vi "Registration with Fourier Mellin Transform.vi"() -> ()   [LabVIEW 2023]
uses:
  <vilib>/vision/NI_Vision_Development_Module.lvlib
panel:
  out "max value (\"Similarity)":sgl
  in  "Images":u16(ring) items=["Shift1-1_Shift1-2", "Shift2-1_Shift2-2"]
  out "DIFF Image":T1(plugin-control)
  out "Inv FFT":T1(plugin-control)
  out "Image 2":T1(plugin-control)
  out "Image 1":T1(plugin-control)
  out "Y Shift":i32
  out "X Shift":i32
  # "Images Registration using Fourier-Mellin Transform"
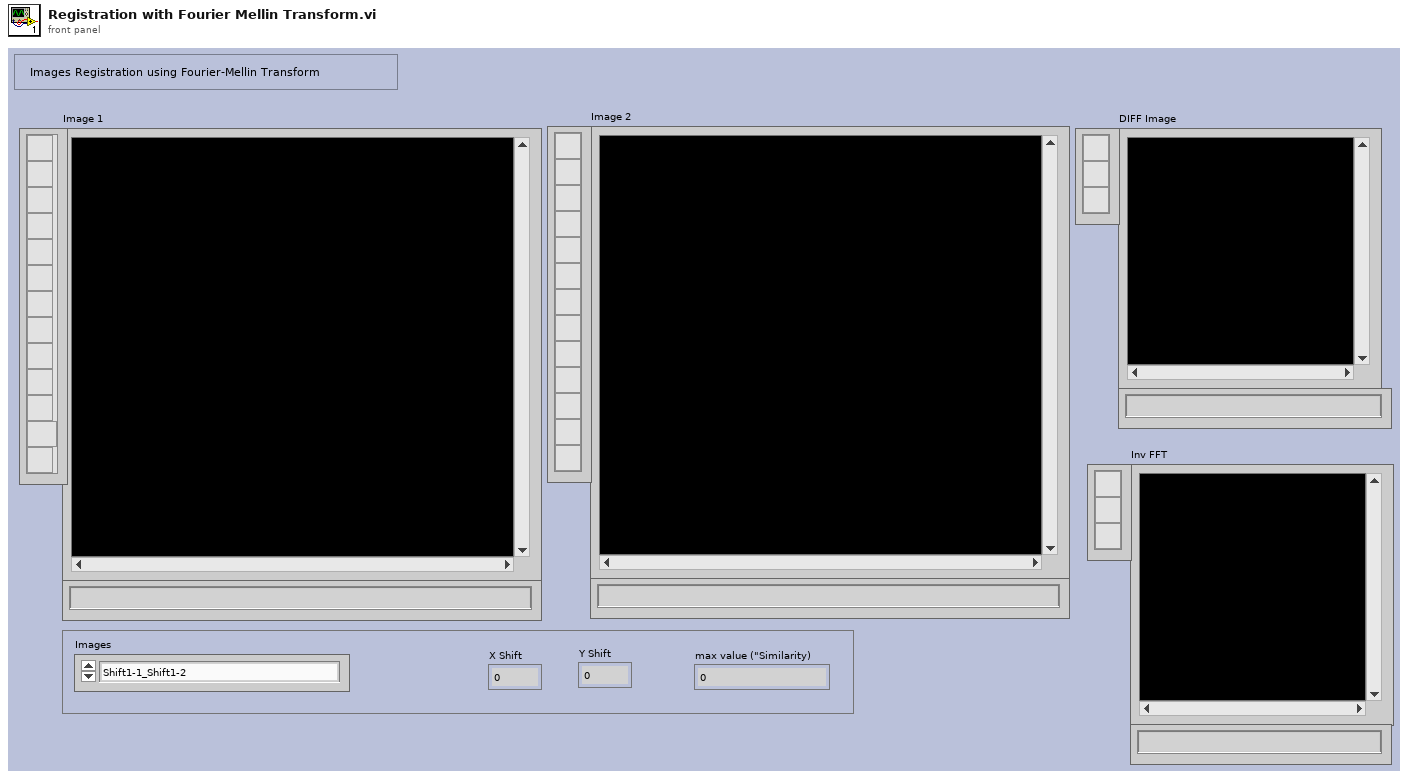
[diagram p1: front panel]
types:
  T1 = typedef "IMAQ Image.ctl" = refnum<image>
  T2 = cluster{"Global Rectangle":i32[], "Contours":cluster{"Contour Type":u32, "ROI Type":u32, "Points":i32[]}[]}
  T3 = typedef "Image Type" = u32
  T4 = typedef "ROI Descriptor" = cluster{"Global Rectangle":i32[], "Contours":cluster{"ID":enum32{"External", "Internal"}, "Type":u32, "Coordinates":i32[]}[]}
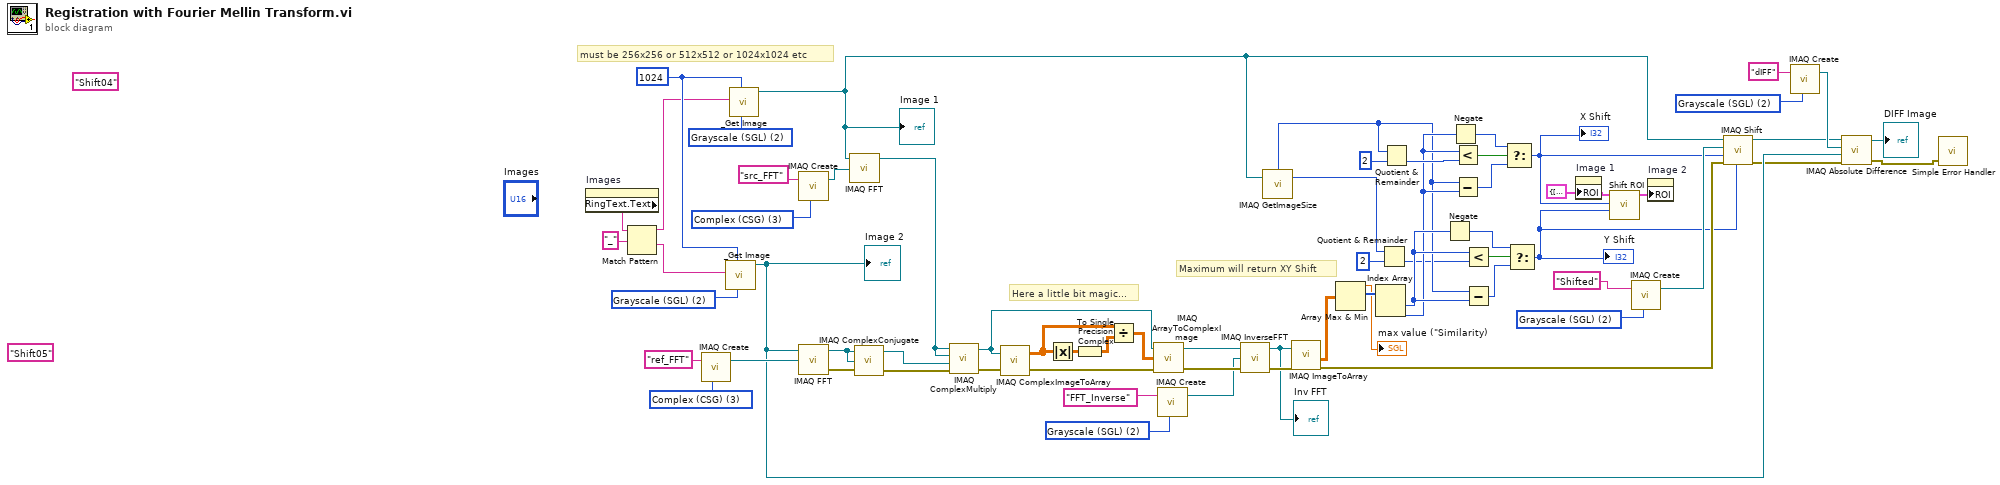
[diagram p0: block diagram]
diagram:
  w5 = T2 {"Global Rectangle"=[344, 290, 717, 642], "Contours"=[{"Contour Type"=0, "ROI Type"=4, "Points"=[404, 335, 668, 593]}, {"Contour Type"=0, "ROI Type"=2, "Points"=[536, 290, 536, 641]}, {"Contour Type"=0, "ROI Type"=2, "Points"=[344, 464, 716, 464]}]} ("ROI")
  w16 = T3 3 items=["Grayscale (U8)", "Grayscale (I16)", "Grayscale (SGL)", "Complex (CSG)", "RGB (U32)", "HSL (U32)", "RGB (U64)", "Grayscale (U16)"] ("Image Type")
  w31 = T3 2 items=["Grayscale (U8)", "Grayscale (I16)", "Grayscale (SGL)", "Complex (CSG)", "RGB (U32)", "HSL (U32)", "RGB (U64)", "Grayscale (U16)"] ("Image Type")
  w32 = T3 3 items=["Grayscale (U8)", "Grayscale (I16)", "Grayscale (SGL)", "Complex (CSG)", "RGB (U32)", "HSL (U32)", "RGB (U64)", "Grayscale (U16)"] ("Image Type")
  w33 = T3 2 items=["Grayscale (U8)", "Grayscale (I16)", "Grayscale (SGL)", "Complex (CSG)", "RGB (U32)", "HSL (U32)", "RGB (U64)", "Grayscale (U16)"] ("Image Type")
  (unwired) "Shift05" ("Image Name")
  (unwired) "Shift04" ("Image Name")
  w20 = 1024 ("XY Resolution")
  w47 = T3 2 items=["Grayscale (U8)", "Grayscale (I16)", "Grayscale (SGL)", "Complex (CSG)", "RGB (U32)", "HSL (U32)", "RGB (U64)", "Grayscale (U16)"] ("Image Type (U16)")
  w48 = T3 2 items=["Grayscale (U8)", "Grayscale (I16)", "Grayscale (SGL)", "Complex (CSG)", "RGB (U32)", "HSL (U32)", "RGB (U64)", "Grayscale (U16)"] ("Image Type (U16)")
  w52 = T3 2 items=["Grayscale (U8)", "Grayscale (I16)", "Grayscale (SGL)", "Complex (CSG)", "RGB (U32)", "HSL (U32)", "RGB (U64)", "Grayscale (U16)"] ("Image Type")
  # "must be 256x256 or 512x512 or 1024x1024 etc"
  # "Maximum will return XY Shift"
  # "Here a little bit magic..."
  n1 = property on="Images" class="Ring (strict)"() -> ("RingText.Text"=w10:string)  [unwired: 2 in, 2 out]
  n2 = Match Pattern(string=w10, regular expression="_") -> (before substring=w8:string, after substring=w7:string)  [unwired: 1 in, 2 out]
  n3 = call "IMAQ Create"("Image Name"="ref_FFT", "Image Type"=w16) -> ("New Image"=w49:T1)  [unwired: 3 in, 1 out]
  n4 = call "_Get Image.vi"("Image Type (U16)"=w47, "XY Resolution"=w20, "Image Name"=w7) -> ("Image Out"=w21:T1)  [unwired: 5 in, 3 out]
  "Image 2" <- w21
  n5 = call "_Get Image.vi"("Image Type (U16)"=w48, "XY Resolution"=w20, "Image Name"=w8) -> ("Image Out"=w18:T1)  [unwired: 5 in, 3 out]
  "Image 1" <- w18
  n6 = call "IMAQ Create"("Image Name"="src_FFT", "Image Type"=w32) -> ("New Image"=w38:T1)  [unwired: 3 in, 1 out]
  n7 = call "IMAQ FFT"("Image Dst"=w49, "Image Src"=w21) -> ("error out"=w23:errorcluster, "Image Dst Out"=w36:T1)  [unwired: 2 in]
  n8 = call "IMAQ FFT"("Image Dst"=w38, "Image Src"=w18) -> ("Image Dst Out"=w37:T1)  [unwired: 2 in, 1 out]
  n9 = call "IMAQ ComplexConjugate"("error in (no error)"=w23, "Image Dst"=w36, "Image Src"=w36) -> ("error out"=w58:errorcluster, "Image Dst Out"=w59:T1)  [unwired: 1 in]
  n10 = call "IMAQ ComplexMultiply"("Image Src A"=w37, "Image Dst"=w37, "Image Src B"=w59, "error in (no error)"=w58) -> ("Image Dst Out"=w64:T1, "error out"=w57:errorcluster)  [unwired: 3 in]
  n11 = call "IMAQ ComplexImageToArray"("Image"=w64, "error in (no error)"=w57) -> ("Image Pixels (Complex)"=w61:csg[][], "error out"=w56:errorcluster)  [unwired: 3 in]
  n12 = Absolute Value(x=w61) -> (abs(x)=w62:sgl[][])
  n13 = To Single Precision Complex(1:w62) -> (0:w66:csg[][])
  n14 = Divide(x=w61, y=w66) -> (x/y=w63:csg[][])
  n15 = call "IMAQ ArrayToComplexImage"("error in (no error)"=w56, "Image Pixels (Complex)"=w63, "Image"=w64) -> ("error out"=w55:errorcluster, "Image Out"=w35:T1)  [unwired: 1 in]
  n16 = call "IMAQ Create"("Image Name"="FFT_Inverse", "Image Type"=w52) -> ("New Image"=w53:T1)  [unwired: 3 in, 1 out]
  n17 = call "IMAQ InverseFFT"("error in (no error)"=w55, "Image Dst"=w53, "Image Src"=w35) -> ("error out"=w54:errorcluster, "Image Dst Out"=w46:T1)  [unwired: 1 in]
  "Inv FFT" <- w46
  n18 = call "IMAQ GetImageSize"("Image"=w18) -> ("Y Resolution"=w14:i32, "X Resolution"=w17:i32)  [unwired: 3 in, 1 out]
  n19 = call "IMAQ ImageToArray"("error in (no error)"=w54, "Image"=w46) -> ("Image Pixels (Float)"=w45:sgl[][], "error out"=w12:errorcluster)  [unwired: 2 in, 3 out]
  n20 = Array Max & Min(array=w45) -> (max value=→"max value (\"Similarity)":sgl, max index (indices)=w65:i32[])  [unwired: 2 out]
  n21 = Index Array(array=w65) -> (element #1=w27:i32, element #2=w26:i32)  [unwired: 2 in]
  n22 = Quotient & Remainder(x=w14, y=2) -> (floor(x/y)=w13:i32)  [unwired: 1 out]
  n23 = Quotient & Remainder(x=w17, y=2) -> (floor(x/y)=w39:i32)  [unwired: 1 out]
  n24 = Negate(x=w27) -> (-x=w24:i32)
  n25 = Negate(x=w26) -> (-x=w25:i32)
  n26 = Less?(x=w26, y=w39) -> (x < y?=w44:bool)
  n27 = Subtract(x=w17, y=w26) -> (x-y=w43:i32)
  n28 = Less?(x=w27, y=w13) -> (x < y?=w41:bool)
  n29 = Subtract(x=w17, y=w27) -> (x-y=w42:i32)
  n30 = Select(t=w25, s=w44, f=w43) -> (s? t:f=w1:i32)
  "X Shift" <- w1
  n31 = Select(t=w24, s=w41, f=w42) -> (s? t:f=w2:i32)
  "Y Shift" <- w2
  n32 = property on="Image 1" class="ImageControl"("ROI"=w5) -> ()  [unwired: 2 in, 2 out]
  n33 = call "Shift ROI.vi"("Y Shift"=w2, "X Shift"=w1, "ROI"=w5) -> ("ROI Descriptor out"=w4:T4)  [unwired: 7 in, 1 out]
  n34 = call "IMAQ Create"("Image Name"="Shifted", "Image Type"=w33) -> ("New Image"=w19:T1)  [unwired: 3 in, 1 out]
  n35 = property on="Image 2" class="ImageControl"("ROI"=w4) -> ()  [unwired: 2 in, 2 out]
  n36 = call "IMAQ Shift"("YOffset"=w2, "error in (no error)"=w12, "XOffset"=w1, "Image Dst"=w19, "Image Src"=w18) -> ("error out"=w11:errorcluster, "Image Dst Out"=w22:T1)  [unwired: 5 in]
  n37 = call "IMAQ Create"("Image Name"="dIFF", "Image Type"=w31) -> ("New Image"=w29:T1)  [unwired: 3 in, 1 out]
  n38 = call "IMAQ Absolute Difference"("Image Src A"=w22, "Image Dst"=w29, "Image Src B"=w21, "error in (no error)"=w11) -> ("Image Dst Out"=→"DIFF Image":T1, "error out"=w3:errorcluster)  [unwired: 3 in]
  n39 = call <vilib>:"Simple Error Handler.vi"("error in (no error)"=w3) -> ()  [unwired: 4 in, 5 out]
